vi "Convert Trigger Position to Phase Difference.vi"(11 "Relative Trigger Position in":dbl[](array[numeric])) -> (3 "Phase Difference":dbl)   [LabVIEW 2024]
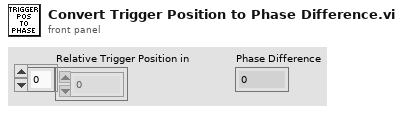
[diagram p1: front panel]
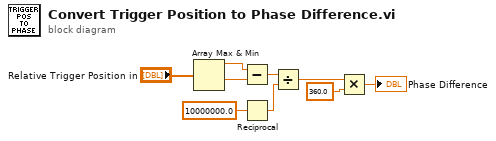
[diagram p0: block diagram]
diagram:
  n1 = Array Max & Min(array="Relative Trigger Position in") -> (max value=w1:dbl, min value=w2:dbl)  [unwired: 2 out]
  n2 = Subtract(x=w1, y=w2) -> (x-y=w7:dbl)
  n3 = Reciprocal(x=10000000.0 ("element")) -> (1/x=w3:dbl)
  n4 = Divide(x=w7, y=w3) -> (x/y=w4:dbl)
  n5 = Multiply(x=w4, y=360.0) -> (x*y=→"Phase Difference":dbl)
